vi "2L03_MIF_extrait_intervalle.vi"(8 "X fin":dbl, 9 "X deb":dbl, 10 "N":dbl[](array[numeric]), 11 "X":dbl[](array[numeric])) -> (0 "i fin":i32, 1 "i deb":i32, 2 "Cumul":dbl, 3 "Nb":i64, 4 "N ds plage":dbl[](array[numeric]), 5 "X_ds plage":dbl[](array[numeric]))   [LabVIEW 2010, in "lv_02.lvlib"]
doc: "X : variable statistique\nY : effectif associé à X\nX deb - X fin représente la plage dans laquelle on va extraire les données de X,N dans \n (X ds Plage) et (N dans Plage)\nNb est le nombre de valeurs trouvées X dans la plage [Xdeb, Xfin[\ni deb et i fin sont les indices de la plage retenue dans le tableau X ou N\nCumul est l'effectif total trouvé dans la plage.\nSi les effectifs N ne sont pas fournis, alors le tableau N est initialisé à 1 pour chaque X"
uses:
  lv_02.lvlib
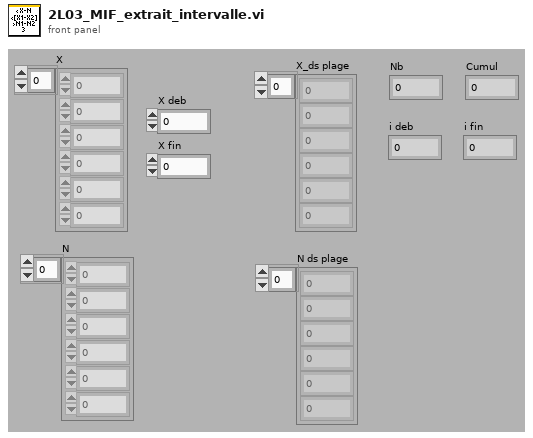
[diagram p1: front panel]
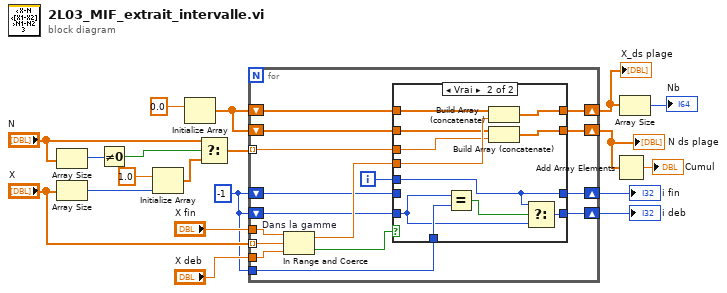
[diagram p0: block diagram]
diagram:
  w1 = -1
  n1 = Array Size(array="N") -> (size(s)=w3:i32)
  n2 = Array Size(array="X") -> (size(s)=w8:i32)
  n3 = Not Equal To 0?(x=w3) -> (x != 0?=w2:bool)
  n4 = Initialize Array(1.0 ("élément"), w8) -> (w7:dbl[])
  n5 = Initialize Array(0.0 ("élément")) -> (w14:dbl[])  [unwired: 1 in]
  n6 = Select(t="N", s=w2, f=w7) -> (s? t:f=w5:dbl[])
  n7 = for {
    tunnel: "X" -> [w33] mode=indexing
    tunnel: "X deb" -> [w35]
    tunnel: "X fin" -> [w34]
    shift-right: [w21] -> w17
    shift-left: w1 -> [w24]
    tunnel: w1 -> [w22]
    shift-right: [w32] -> w13
    shift-left: w14 -> [w30]
    shift-right: [w29] -> w11
    shift-left: w14 -> [w28]
    shift-right: [w26] -> w9
    shift-left: w1 -> [w27]
    tunnel: w5 -> [w23] mode=indexing
    i -> [w25]
    n8 = In Range and Coerce "Dans la gamme"(upper limit=w34, x=w33, lower limit=w35) -> (coerced(x)=w31:dbl, In Range?=w20:bool)
    n9 = case shown="Vrai" w20 {
      tunnel: [w39 w50] -> w32
      tunnel: w31 -> [_ w49]
      tunnel: w30 -> [w39 w48]
      tunnel: [w37 w47] -> w29
      tunnel: w23 -> [_ w46]
      tunnel: w28 -> [w37 w45]
      tunnel: w27 -> [w38 _]
      tunnel: [w38 w42] -> w26
      tunnel: w25 -> [_ w42]
      tunnel: w24 -> [w36 w41]
      tunnel: w22 -> [_ w44]
      tunnel: [w36 w40] -> w21
      frame False {
      }
      frame True {
        n10 = Equal?(x=w41, y=w44) -> (x = y?=w43:bool)
        n11 = Build Array (concatenate)(w48, w49) -> (w50:dbl[])
        n12 = Build Array (concatenate)(w45, w46) -> (w47:dbl[])
        n13 = Select(t=w42, s=w43, f=w41) -> (s? t:f=w40:i32)
      }
    }
  }
  "X_ds plage" <- w13
  "i deb" <- w17
  "i fin" <- w9
  "N ds plage" <- w11
  n14 = Add Array Elements(numeric array=w11) -> (sum=→"Cumul":dbl)
  n15 = Array Size(array=w13) -> (size(s)=→"Nb":i32)
